vi "Invalid Type.vi"() -> ()   [LabVIEW 2017, in "Transparent Assertions.Tests.lvlib" / "Assert Not Refnum.lvlib"]
uses:
  Assert Not Refnum.lvlib
  src/Transparent Assertions/Transparent Assertions.lvlib
panel:
  out "error out":errorcluster
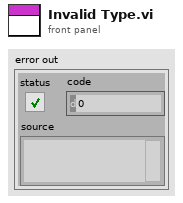
[diagram p1: front panel]
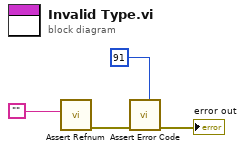
[diagram p0: block diagram]
diagram:
  n1 = call "Assert Refnum.vi"("Refnum"="") -> ("error out"=w4:errorcluster)  [unwired: 10 in]
  n2 = call "Assert Error Code.vi"("Expected"=91, "error in (no error)"=w4) -> ("error out"=→"error out":errorcluster)  [unwired: 9 in]
